vi "Protocol Settings.vi"() -> (2 "Frame sync clock control":T1, 3 "PDM data configuration":T3)   [LabVIEW 2021, in "Audio ADC Shared.lvlib"]
uses:
  Audio ADC Shared.lvlib
  <vilib>/PDM Acquisition Toolkit/shared/controls/PCM Data Format Configuration.ctl
  <vilib>/PDM Acquisition Toolkit/shared/controls/Digital Edge.ctl
  <vilib>/PDM Acquisition Toolkit/shared/controls/PCM Bit Endianness.ctl
  <vilib>/PDM Acquisition Toolkit/shared/controls/PCM Data Justification.ctl
  <vilib>/PDM Acquisition Toolkit/shared/controls/PCM Frame Sync Control.ctl
  controls/PCM Interface Type_Copy.ctl
  <vilib>/PDM Acquisition Toolkit/shared/PDM Shared.lvlib
  controls/Audio ADC Controls.lvlib
panel:
  in  "TDM":bool
  in  "RJ":bool
  in  "LJ":bool
  in  "I2S":bool
  in  "Bit clock edge  sync":enum8{"Rising", "Falling"}(ring)=enum."Falling"
  in  "Frame sync pulse width":u16=32
  in  "Frame length":u16=64
  in  "Data Justification":enum16{"Left Justified", "Right Justified"}(ring) caption="Data justification"
  in  "Endianness":enum16{"MSB First", "LSB First"}(ring)
  in  "Channel 0 offset":u16=1
  in  "Bit depth":u8=24
  in  "Channel length":u16=32
  in  "Channel count per frame":u8=2
  in  "Frame sync edge for Channel 0":enum16{"Rising", "Falling"}(ring)=enum."Falling"
  # "Protocols"
  # "PCM data configuration"
  # "Frame sync clock control"
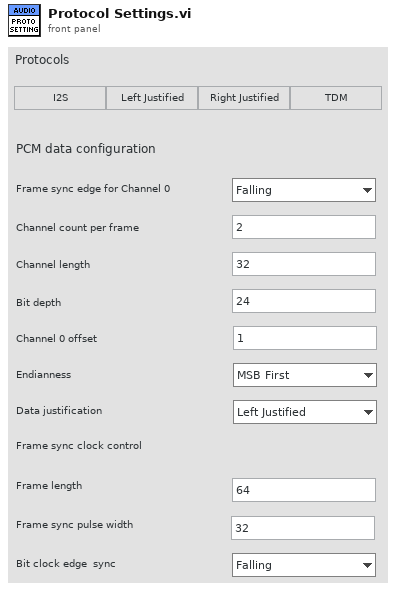
[diagram p1: front panel]
types:
  T1 = typedef "PDM Shared.lvlib/PCM Frame Sync Control.ctl" = cluster{"Frame Length":u16, "Frame Sync Pulse Width":u16, "Bit Clock Edge  Sync":T2}
  T2 = typedef "PDM Shared.lvlib/Digital Edge.ctl" = enum8{"Rising", "Falling"}
  T3 = typedef "PDM Shared.lvlib/PCM Data Format Configuration.ctl" = cluster{"Frame Sync Edge for Channel 0":T2, "Channel Count Per Frame":u8, "Channel Length":u16, "Bit Depth":u8, "Channel 0 Offset":u16, "Endianness":T4, "Data Justification":T5}
  T4 = typedef "PDM Shared.lvlib/PCM Bit Endianness.ctl" = enum16{"MSB First", "LSB First"}
  T5 = typedef "PDM Shared.lvlib/PCM Data Justification.ctl" = enum16{"Left Justified", "Right Justified"}
  T6 = enum32{"Invalid", "Standard", "Closed", "Hidden", "Minimized", "Maximized"}
  T7 = typedef "Audio ADC Controls.lvlib/PCM Interface Type_Copy.ctl" = enum16{"I2S", "Left Justified", "Right Justified", "TDM 4 Channel", "TDM 6 Channel", "TDM 8 Channel", "DSP mode", "DSP mode with 1 bit delay", "PCM Short Frame", "PCM Long Frame"}
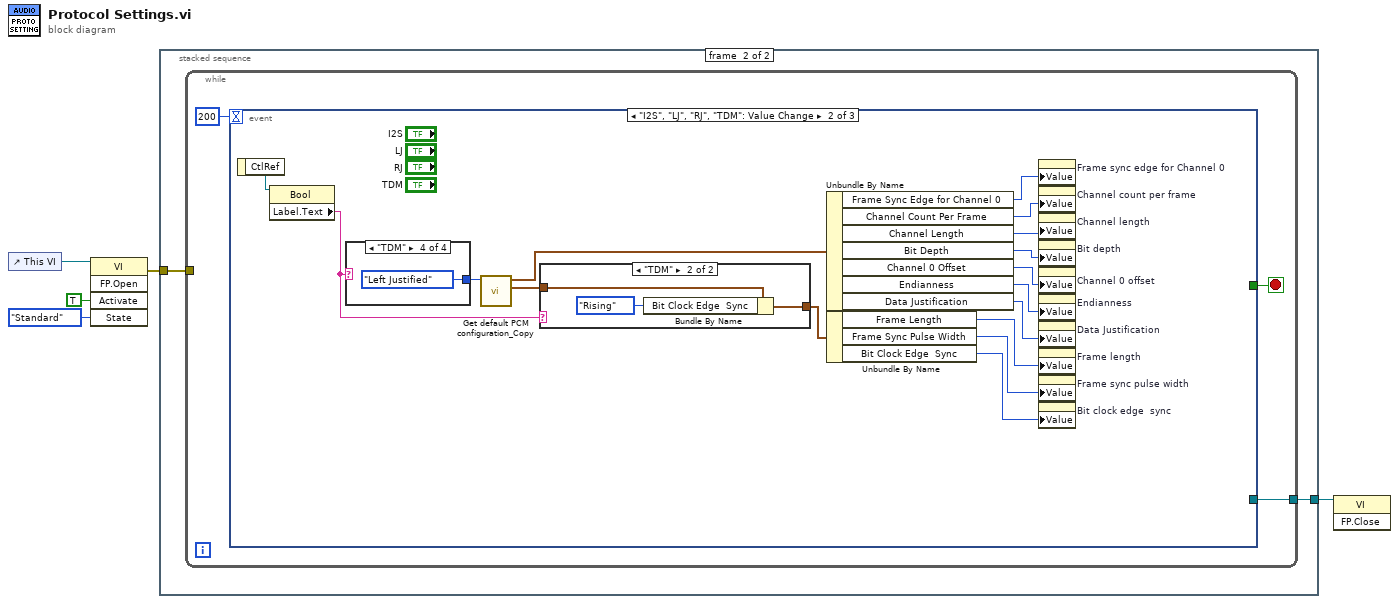
[diagram p0: block diagram]
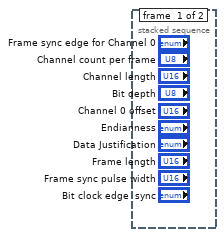
[diagram p2: hidden frame]
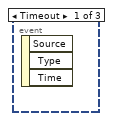
[diagram p3: hidden frame]
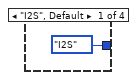
[diagram p5: hidden frame]
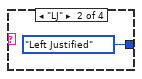
[diagram p6: hidden frame]
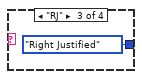
[diagram p7: hidden frame]
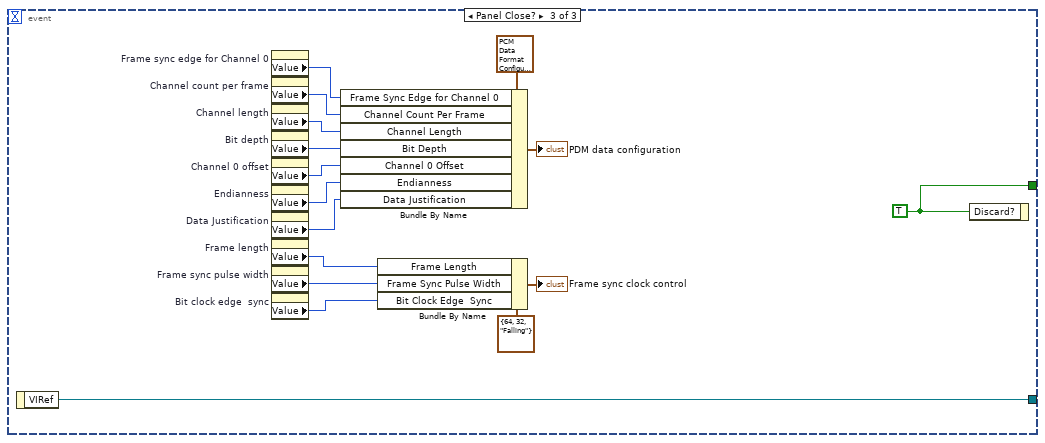
[diagram p8: hidden frame]
diagram:
  n1 = control-ref of="This VI"() -> (w3:refnum<vi>)
  n2 = invoke class="VI" method="FP.Open"(reference=w3, "Activate"=TRUE ("Activate?"), "State"=T6."Standard") -> (error out=w2:errorcluster)  [unwired: 2 in, 4 out]
  n3 = stacked-sequence {
    tunnel: w2 -> [_ w7]
    tunnel: [_ w6] -> w1
    frame #0 {
    }
    frame #1 {
      n4 = while {
        tunnel: [w8] -> w6
        tunnel: w7 -> [_]
        stop <- w10 stop-if-true
        n5 = event shown="[1] \"I2S\", \"LJ\", \"RJ\", \"TDM\": Value Change" {
          selector: _ -> [_ _ _]
          dyn-events: _ -> [_ _ _]
          timeout: 200 -> [_ _ _]
          tunnel: [_ _ w42] -> w10
          tunnel: [_ _ w43] -> w8
          event Timeout {
            n6 = event-data() -> ()  [unwired: 1 in, 3 out]
          }
          event "I2S", "LJ", "RJ", "TDM": Value Change {
            n7 = event-data() -> ("CtlRef"=w15:refnum<vi>)  [unwired: 1 in]
            n8 = property class="Bool"(reference=w15) -> ("Label.Text"=w14:string)  [unwired: 1 in, 2 out]
            n9 = case shown="\"TDM\"" w14 {
              tunnel: [PCM_Interface_Type_Copy."I2S" ("PCM Interfaces") PCM_Interface_Type_Copy."Left Justified" ("PCM Interfaces") PCM_Interface_Type_Copy."Right Justified" ("PCM Interfaces") PCM_Interface_Type_Copy."Left Justified" ("PCM Interfaces")] -> w26
              frame "I2S", Default {
              }
              frame "LJ" {
              }
              frame "RJ" {
              }
              frame "TDM" {
              }
            }
            n10 = call "Get default PCM configuration_Copy.vi"("PCM Interfaces"=w26) -> ("Frame Sync Clock Control"=w13:T1, "PCM Data Configuration"=w11:T3)  [unwired: 9 in]
            n11 = case shown="\"TDM\"" w14 {
              tunnel: w13 -> [w27 w30]
              tunnel: [w27 w28] -> w12
              frame "I2S", Default {
              }
              frame "TDM" {
                n12 = Bundle By Name(cluster=w30, "Bit Clock Edge  Sync"=Digital_Edge."Rising") -> (w28:T1)
              }
            }
            n13 = Unbundle By Name(w11) -> ("Frame Sync Edge for Channel 0"=w16:T2, "Channel Count Per Frame"=w17:u8, "Channel Length"=w18:u16, "Bit Depth"=w19:u8, "Channel 0 Offset"=w20:u16, "Endianness"=w21:T4, "Data Justification"=w22:T5)
            n14 = Unbundle By Name(w12) -> ("Frame Length"=w23:u16, "Frame Sync Pulse Width"=w24:u16, "Bit Clock Edge  Sync"=w25:T2)
            n15 = property on="Frame sync edge for Channel 0" class="Enum (strict)"("Value"=w16) -> ()  [unwired: 2 in, 2 out]
            n16 = property on="Channel count per frame" class="DigNum (strict)"("Value"=w17) -> ()  [unwired: 2 in, 2 out]
            n17 = property on="Channel length" class="DigNum (strict)"("Value"=w18) -> ()  [unwired: 2 in, 2 out]
            n18 = property on="Bit depth" class="DigNum (strict)"("Value"=w19) -> ()  [unwired: 2 in, 2 out]
            n19 = property on="Channel 0 offset" class="DigNum (strict)"("Value"=w20) -> ()  [unwired: 2 in, 2 out]
            n20 = property on="Endianness" class="Enum (strict)"("Value"=w21) -> ()  [unwired: 2 in, 2 out]
            n21 = property on="Data Justification" class="Enum (strict)"("Value"=w22) -> ()  [unwired: 2 in, 2 out]
            n22 = property on="Frame length" class="DigNum (strict)"("Value"=w23) -> ()  [unwired: 2 in, 2 out]
            n23 = property on="Frame sync pulse width" class="DigNum (strict)"("Value"=w24) -> ()  [unwired: 2 in, 2 out]
            n24 = property on="Bit clock edge  sync" class="Enum (strict)"("Value"=w25) -> ()  [unwired: 2 in, 2 out]
          }
          event Panel Close? {
            w42 = TRUE ("Discard?")
            n25 = event-data() -> ("VIRef"=w43:refnum<vi>)  [unwired: 1 in]
            n26 = property on="Frame sync edge for Channel 0" class="Enum (strict)"() -> ("Value"=w50:enum16{"Rising", "Falling"})  [unwired: 2 in, 2 out]
            n27 = property on="Channel count per frame" class="DigNum (strict)"() -> ("Value"=w49:u8)  [unwired: 2 in, 2 out]
            n28 = property on="Channel length" class="DigNum (strict)"() -> ("Value"=w48:u16)  [unwired: 2 in, 2 out]
            n29 = property on="Bit depth" class="DigNum (strict)"() -> ("Value"=w47:u8)  [unwired: 2 in, 2 out]
            n30 = property on="Channel 0 offset" class="DigNum (strict)"() -> ("Value"=w44:u16)  [unwired: 2 in, 2 out]
            n31 = property on="Endianness" class="Enum (strict)"() -> ("Value"=w46:enum16{"MSB First", "LSB First"})  [unwired: 2 in, 2 out]
            n32 = property on="Data Justification" class="Enum (strict)"() -> ("Value"=w45:enum16{"Left Justified", "Right Justified"})  [unwired: 2 in, 2 out]
            n33 = property on="Frame length" class="DigNum (strict)"() -> ("Value"=w36:u16)  [unwired: 2 in, 2 out]
            n34 = property on="Frame sync pulse width" class="DigNum (strict)"() -> ("Value"=w38:u16)  [unwired: 2 in, 2 out]
            n35 = property on="Bit clock edge  sync" class="Enum (strict)"() -> ("Value"=w37:enum8{"Rising", "Falling"})  [unwired: 2 in, 2 out]
            n36 = Bundle By Name(cluster=T3 {"Frame Sync Edge for Channel 0"=enum."Falling", "Channel Count Per Frame"=2, "Channel Length"=32, "Bit Depth"=24, "Channel 0 Offset"=1, "Endianness"=enum."MSB First", "Data Justification"=enum."Left Justified"} ("PCM Data Configuration"), "Frame Sync Edge for Channel 0"=w50, "Channel Count Per Frame"=w49, "Channel Length"=w48, "Bit Depth"=w47, "Channel 0 Offset"=w44, "Endianness"=w46, "Data Justification"=w45) -> (→"PDM data configuration":T3)
            n37 = Bundle By Name(cluster=T1 {"Frame Length"=64, "Frame Sync Pulse Width"=32, "Bit Clock Edge  Sync"=enum."Falling"} ("Frame Sync Clock Control"), "Frame Length"=w36, "Frame Sync Pulse Width"=w38, "Bit Clock Edge  Sync"=w37) -> (→"Frame sync clock control":T1)
            n38 = event-data("Discard?"=w42) -> ()  [unwired: 1 in, 1 out]
          }
        }
      }
    }
  }
  n39 = invoke class="VI" method="FP.Close"(reference=w1) -> ()  [unwired: 2 in, 3 out]
